vi "SetMaxDrivingPower.vi"(9 "Reinit":bool, 10 "HMI to Control":T1, 11 "SensorInputData":T5) -> (2 "HMI to ControlOut":T1, 3 "SensorInputDataOut":T5, 4 "Done":bool=TRUE)   [LabVIEW 2014]
uses:
  Typedefs/SensorInputData.ctl
  Typedefs/HMI_to_Control.ctl
  Typedefs/Arm States.ctl
  Typedefs/ClawStates.ctl
  Typedefs/IntakeWheelSenseOrManual.ctl
  Gensubs/Maximum Power Allowed.vi
panel:
  in  "arguments":string[](array[string])
  in  "dt":i32
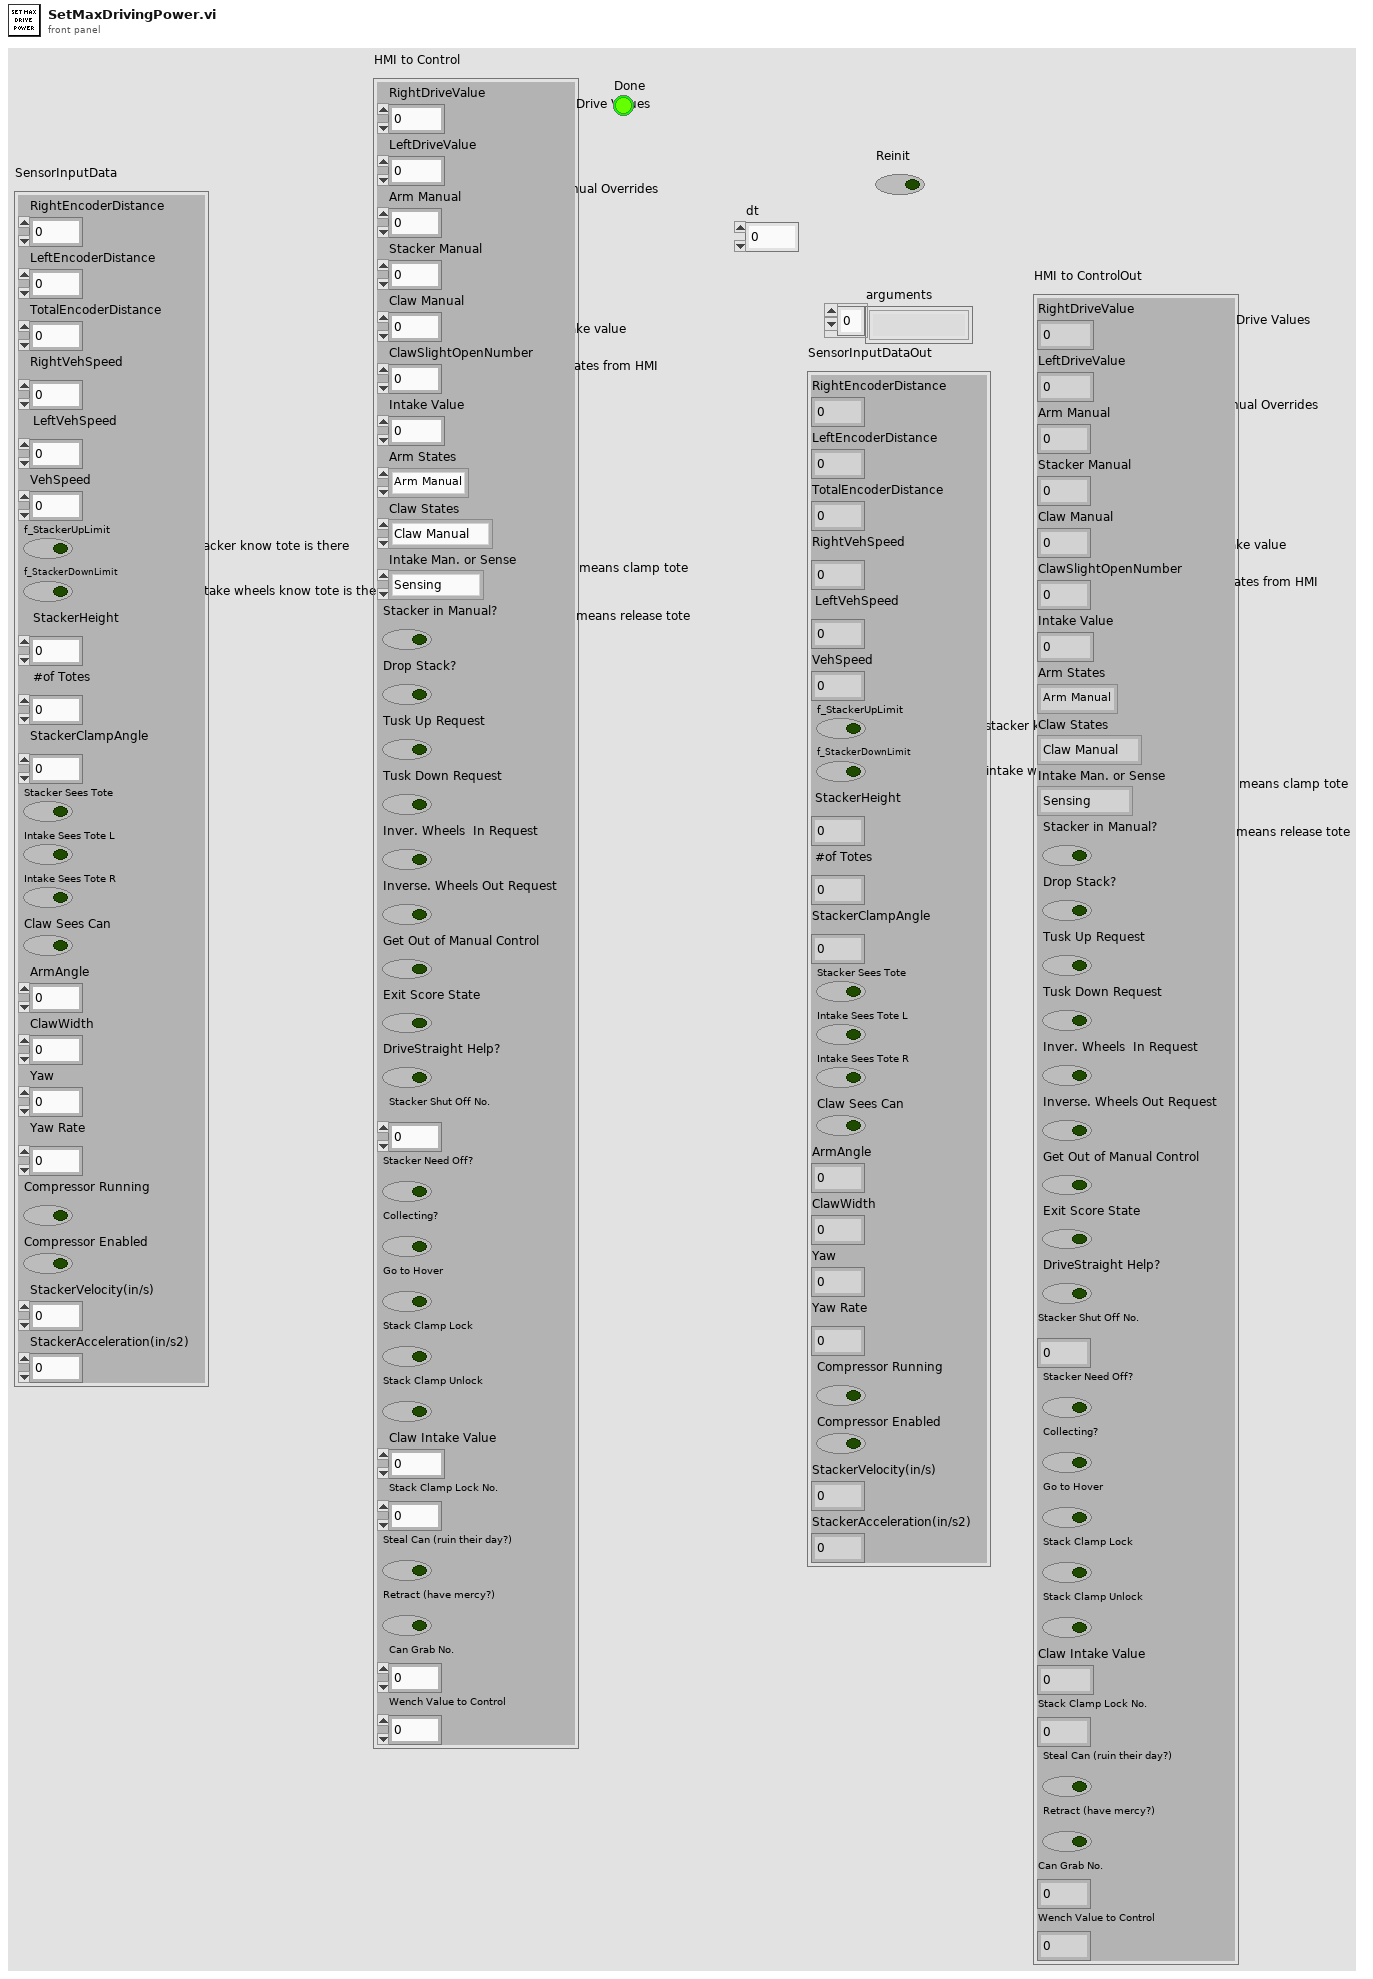
[diagram p1: front panel]
types:
  T1 = typedef "HMI_to_Control.ctl" = cluster{"RightDriveValue":dbl, "LeftDriveValue":dbl, "Arm Manual ":dbl, "Stacker Manual ":dbl, "Claw Manual ":dbl, "ClawSlightOpenNumber":i8, "Intake Value ":sgl, "Arm States":T2, "Claw States":T3, "Intake Man. or Sense":T4, "Stacker in Manual?":bool, "Drop Stack? ":bool, "Tusk Up Request":bool, "Tusk Down Request":bool, "Inver. Wheels  In Request":bool, "Inverse. Wheels Out Request ":bool, "Get Out of Manual Control":bool, "Exit Score State":bool, "DriveStraight Help?":bool, "Stacker Shut Off No.":i8, "Stacker Need Off?":bool, "Collecting?":bool, "Go to Hover":bool, "Stack Clamp Lock ":bool, "Stack Clamp Unlock ":bool, "Claw Intake Value ":sgl, "Stack Clamp Lock No. ":i8, "Steal Can (ruin their day?)":bool, "Retract (have mercy?)":bool, "Can Grab No. ":i8, "Wench Value to Control ":dbl}
  T2 = typedef "Arm States.ctl" = enum16{"Arm Manual ", "Ground", "Step", "1 Tote", "2 Tote", "3 Tote", "4 Tote", "5 Tote", "6 Tote", "Flip Can Arm", "Grab Can in auto", "Nudge"}
  T3 = typedef "ClawStates.ctl" = enum16{"Claw Manual ", "Claw Open", "Claw Closed", "Claw Slight Open", "Flip Can"}
  T4 = typedef "IntakeWheelSenseOrManual.ctl" = enum16{"Sensing", "Manual "}
  T5 = typedef "SensorInputData.ctl" = cluster{"RightEncoderDistance":dbl, "LeftEncoderDistance":dbl, "TotalEncoderDistance":dbl, "RightVehSpeed":dbl, "LeftVehSpeed":dbl, "VehSpeed":dbl, "f_StackerUpLimit":bool, "f_StackerDownLimit":bool, "StackerHeight":dbl, "#of Totes":u8, "StackerClampAngle":dbl, "Stacker Sees Tote":bool, "Intake Sees Tote L":bool, "Intake Sees Tote R":bool, "Claw Sees Can":bool, "ArmAngle":dbl, "ClawWidth":dbl, "Yaw":dbl, "Yaw Rate":dbl, "Compressor Running":bool, "Compressor Enabled":bool, "StackerVelocity(in/s)":dbl, "StackerAcceleration(in/s2)":dbl}
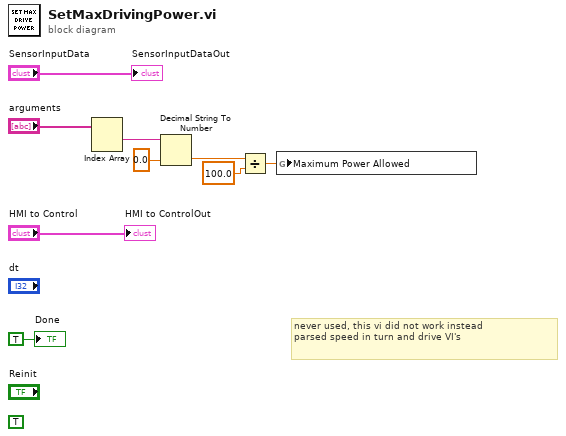
[diagram p0: block diagram]
diagram:
  (unwired) TRUE ("Inver. Wheels  In Request")
  # "never used, this vi did not work instead \nparsed speed in turn and drive VI's"
  n1 = Index Array(array="arguments") -> (element #1=w5:string)  [unwired: 2 in, 1 out]
  n2 = Decimal String To Number(string=w5, default (0L)=0.0) -> (number=w3:dbl)  [unwired: 1 in, 1 out]
  n3 = Divide(x=w3, y=100.0) -> (x/y=w1:dbl)
  n4 = global write "Maximum Power Allowed.vi" "Maximum Power Allowed"(w1) -> ()
  "SensorInputDataOut" <- "SensorInputData"
  "HMI to ControlOut" <- "HMI to Control"
  "Done" <- TRUE
